vi "VI Anlagenuebersicht.vi"() -> (3 "XML-String":string)   [LabVIEW 2020, in "Anlagenuebersicht.lvlib"]
uses:
  VisBx Anzeige/Anlagenuebersicht.lvlib
  VisBx Anzeige/Messwerte.ctl
  PNS/Aktionen FGV Grenzwerte.ctl
  cRIO/PC/Kommunikation mit cRIO.lvlib
  Funktionstasten/Funktionstasten.lvlib
  Funktionstasten/Funktionstasten-Aktion.ctl
  Funktionstasten/Zustaende.ctl
  CalGas Aufschaltung/Auswahl Aufschaltpunkt.ctl
  CalGas Aufschaltung/CalGas Aufschaltung.lvlib
  CalGas Aufschaltung/FGV CalGas Aktionen.ctl
  PNS/PNS.lvlib
  PNS/Aktionen FGV Istwerte.ctl
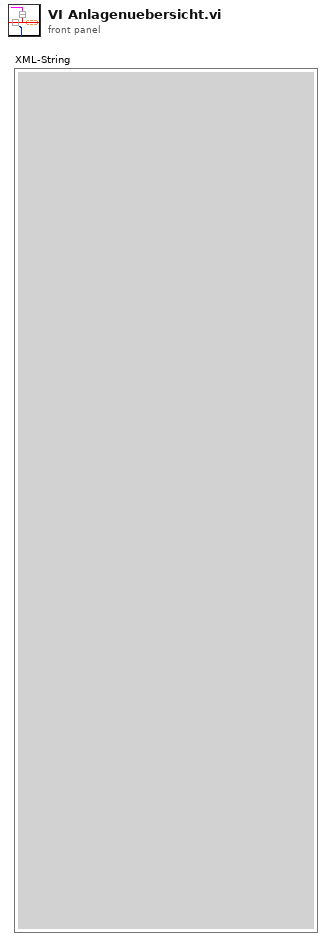
[diagram p1: front panel]
types:
  T1 = enum16{"Stby/Pause/Eco", "Messen", "Spülen Filter", "Spülen Leitung", "Umgebungsluft", "0-Gas / Hintergrund", "Cal-Gas"}
  T2 = typedef "Anlagenuebersicht.lvlib/Messwerte.ctl" = cluster{"-17S1":bool, "-17S2":bool, "-17S5":bool, "-17S6":bool, "-18B6":bool, "-16B1":bool, "-16B2":bool, "DI Reserve 1":bool, "DI Reserve 2":bool, "DI Reserve 3":bool, "DI Reserve 4":bool, "DI Reserve 5":bool, "-20Y1":bool, "-20Y2":bool, "-20Y3":bool, "-20Y4":bool, "-20Y5":bool, "-20Y6":bool, "-20Y7":bool, "-20Y8":bool, "-21Y1":bool, "-21Y2":bool, "-21Y3":bool, "-21Y4":bool, "-21Y5":bool, "-21Y6":bool, "-21Y7":bool, "-21Y8":bool, "-22Y1":bool, "-22Y2":bool, "-22Y3":bool, "-22Y4":bool, "-22Y5":bool, "-22Y6":bool, "-22Y7":bool, "-23Y1":bool, "-23Y2":bool, "-23Y3":bool, "-23Y4":bool, "-23Y5":bool, "-23Y6":bool, "-23Y7":bool, "Messgaspumpe EIN":bool, "Absaugung EIN":bool, "Kompressor":bool, "-23Y8":bool, "-11Y2":bool, "-11Y3":bool, "-11Y5":bool, "-11Y6":bool, "-11Y7":bool, "-11Y8":bool, "-12Y1":bool, "Zustand":enum16{"Stby/Pause/Eco", "Messen", "Spülen Filter", "Spülen Leitung", "Umgebungsluft", "0-Gas / Hintergrund", "Cal-Gas"}, "Reserve 1":bool, "Reserve 2":bool, "Reserve 3":bool, "Reserve 4":bool, "Reserve 5":bool, "Reserve 6":bool, "Reserve 7":bool, "Reserve 8":bool, "Reserve 9":bool, "Reserve 10":bool, "Reserve 11":bool, "Reserve 12":bool, "Reserve 13":bool, "Reserve 14":bool, "Reserve 15":bool, "Reserve 16":bool}
  T3 = typedef "CalGas Aufschaltung.lvlib/FGV CalGas Aktionen.ctl" = enum16{"lesen", "Analysator Auswahl", "Def.CalGas", "Aufschaltung CalGas", "laden", "speichern", "KAL extrahieren"}
  T4 = typedef "Funktionstasten.lvlib/Zustaende.ctl" = enum16{"Standby", "Pause", "Eco", "Messen", "Kalibrieren", "Spülen Filter", "Spülen Leitung", "Umgebungsluft", "0-Gas", "Cal-Gas", "CG zu PNS", "-------------", "Init 1", "Init 2", "Init 3", "Init 4", "Messen vorbereiten", "Messen durchführen", "Exit"}
  T5 = typedef "CalGas Aufschaltung.lvlib/Auswahl Aufschaltpunkt.ctl" = enum16{"über Filterblock", "Analysator direkt", "über PNS", "Entnahme", "Gasdivider"}
  T6 = typedef "Funktionstasten.lvlib/Funktionstasten-Aktion.ctl" = enum16{"Initialisieren", "Zustand setzen", "Taste gedrückt", "Fehler speichern", "Lesen", "Manuell", "Remote", "Bitparallel", "Samplepoint", "Zeit Prüfen", "reset Umschalten"}
  T7 = typedef "CalGas Aufschaltung.lvlib/Aufschaltung CalGas.ctl" = cluster{"Kalibriergas":T8, "Aufschaltpunkt":T5, "Analysator":T9}
  T8 = typedef "Auswahlfeld.ctl" = u16
  T9 = typedef "CalGas Aufschaltung.lvlib/Auswahl Analysator.ctl" = enum16{"FT-IR", "FID", "PMA", "PMA/FID/FT-IR"}
  T10 = typedef "PNS.lvlib/Aktionen FGV Istwerte.ctl" = enum16{"lesen", "initialisieren", "schreiben", "Störungen"}
  T11 = typedef "PNS.lvlib/Aktionen FGV Grenzwerte.ctl" = enum16{"lesen", "Grenzw. schreiben", "Anweisungscode", "IP-Adresse", "laden", "speichern", "Anweisungscode vorgeben"}
  T12 = typedef "Verwaltung - cRIO.lvlib/Digital Eingaenge 0-15.ctl" = cluster{"I0: N2 Nachf. FT-IR voll":bool, "I1: N2 Nachf. Vorrat leer":bool, "I2: (Klimaanlage eingeschaltet)":bool, "I3: (Klimaanlage Störung)":bool, "I4: Trigger Eingang (Messdaten sp.)":bool, "I5: Reserve":bool, "I6: Reserve":bool, "I7: Reserve":bool, "I8: Druckschalter Versorgung ok":bool, "I9: Reserve":bool, "I10: Reserve":bool, "I11: Reserve":bool, "I12: Drucksch. N2 Versorgung":bool, "I13: Reserve":bool, "I14: Drucksch. N2 Optikbox":bool, "I15: (Füllstand Kondensatbehälter)":bool}
  T13 = typedef "Verwaltung - cRIO.lvlib/Digital Ausgaenge 0-31.ctl" = cluster{"O0: Druckluft Versorgung":bool, "O1: CG 1 (FB Eingang 1)":bool, "O2: CG 2 (Kühlung FT-IR EIN)":bool, "O3: CG 3 (FB Bypass)":bool, "O4: CG 4 (FB CalGas)":bool, "O5: CG 5 (FB spülen/UL)":bool, "O6: CG 6 (FB zum FT-IR)":bool, "O7: CG 7 (FB zum FID)":bool, "O8: CG 8 (FB Reserve)":bool, "O9: (FB Reserve)":bool, "O10: (FB Umgebungsluft FID)":bool, "O11: (FB zum Gaskühler)":bool, "O12: FB Stickstoff zu FT-IR":bool, "O13: Optikbox FT-IR spülen":bool, "O14: (Purifier deaktivieren)":bool, "O15: (Umschaltung Purifier/Stickstoff)":bool, "O16: N2 Einblasung":bool, "O17: LSP LN2 Nachfüllung":bool, "O18: (Reserve)":bool, "O19: (Pumpe Eingang1)":bool, "O20: (Pumpe Eingang2)":bool, "O21: (Pumpe Spülen1)":bool, "O22: (Pumpe Spülen2)":bool, "O23: (Reserve)":bool, "O24: CalGas 1":bool, "O25: CalGas 2":bool, "O26: CG 3-8 (CalGas 3)":bool, "O27: Stickstoff aufschalten":bool, "O28: CG zu PNS":bool, "O29: FTIR Standby Spülung":bool, "O30: CG zu Entnahme(T90)":bool, "O31: (Purifier regenerieren)":bool}
  T14 = typedef "Verwaltung - cRIO.lvlib/Digital Ausgaenge 32-63.ctl" = cluster{"O32: Messgaspumpe EIN":bool, "O33: (Umgebungsluftpumpe)":bool, "O34: (Kondensatpumpe GK)":bool, "O35: Klima/Lüfter EIN":bool, "O36: Versorgung Heizungen":bool, "O37: Versorgung Heizungen":bool, "O38: (Gaskühler EIN (Freigabe))":bool, "O39: Störung FAS LP":bool, "O40: (Heizung Filterblock)":bool, "O41: Heizung HL zu FT-IR":bool, "O42: Heizung HL Extern SP1":bool, "O43: Heizung HL Extern SP2":bool, "O44: Heizung Reserve":bool, "O45: Heizung Reserve":bool, "O46: Statusbeleuchtung grün":bool, "O47: Statusbeleuchtung rot":bool}
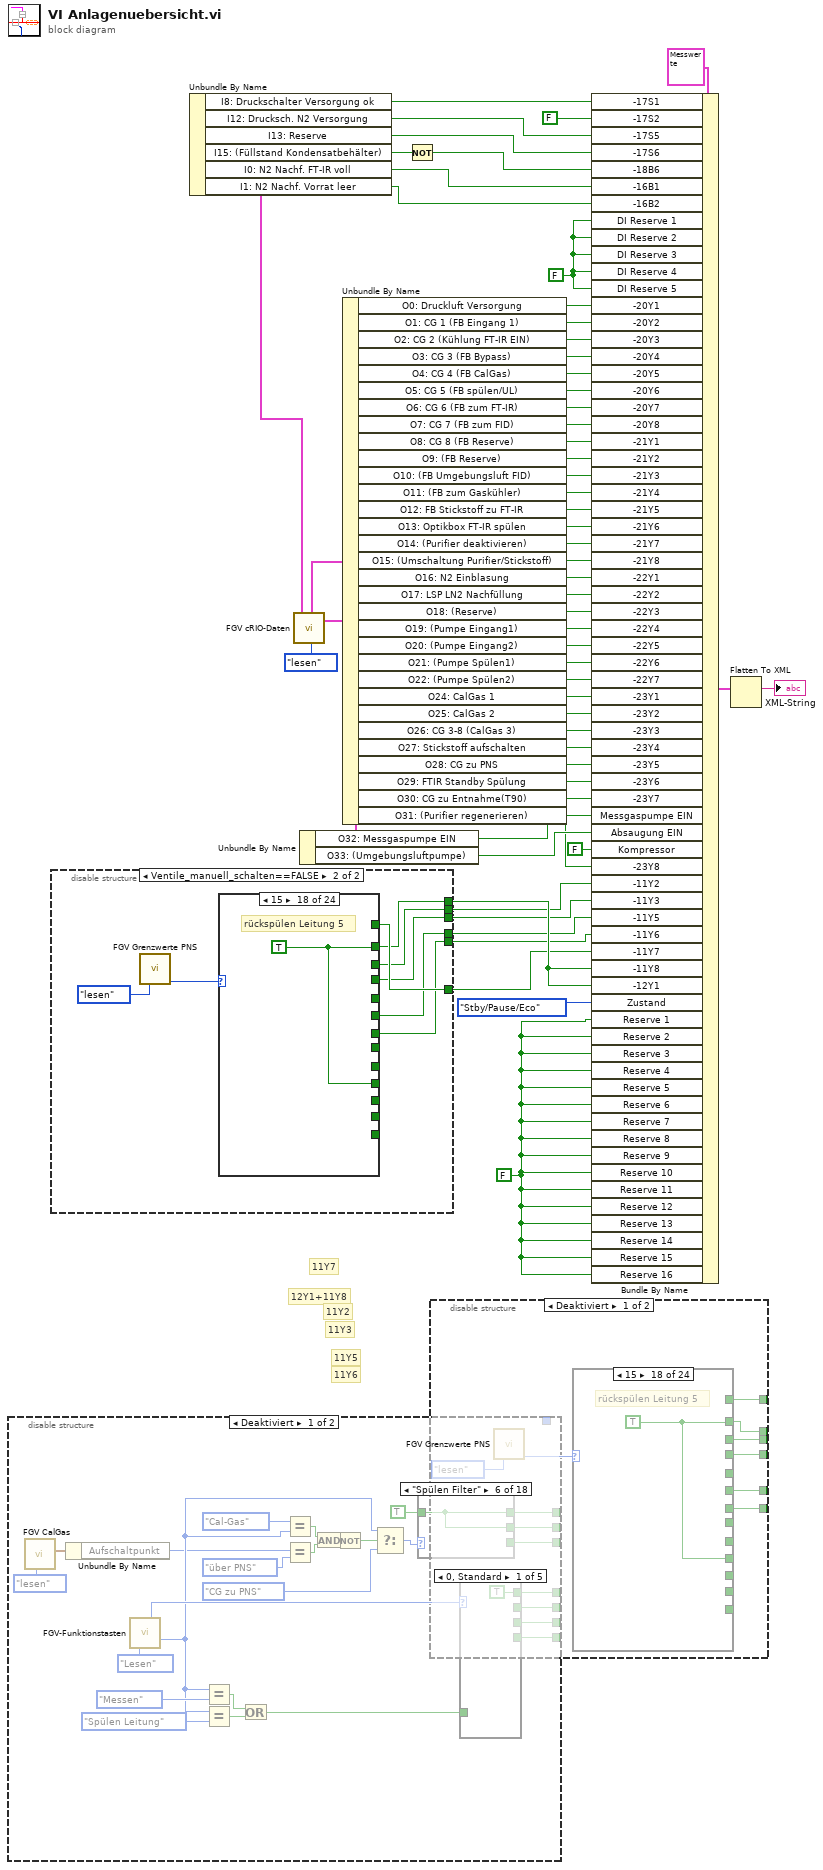
[diagram p0: block diagram]
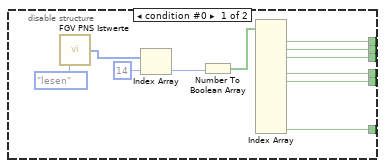
[diagram p2: hidden frame]
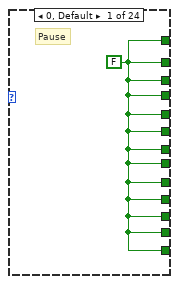
[diagram p3: hidden frame]
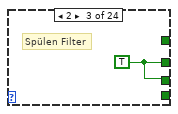
[diagram p5: hidden frame]
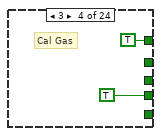
[diagram p6: hidden frame]
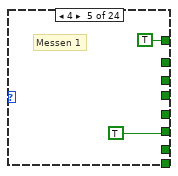
[diagram p7: hidden frame]
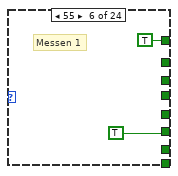
[diagram p8: hidden frame]
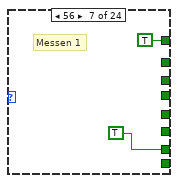
[diagram p9: hidden frame]
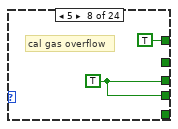
[diagram p10: hidden frame]
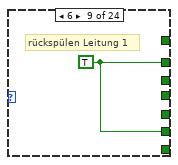
[diagram p11: hidden frame]
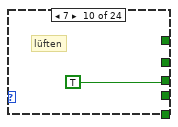
[diagram p12: hidden frame]
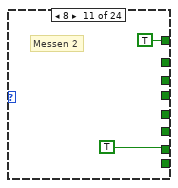
[diagram p13: hidden frame]
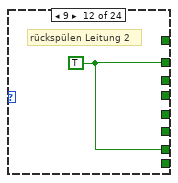
[diagram p14: hidden frame]
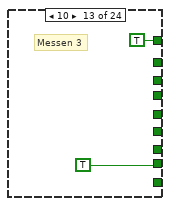
[diagram p15: hidden frame]
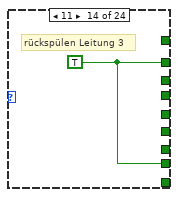
[diagram p16: hidden frame]
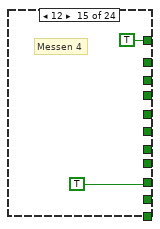
[diagram p17: hidden frame]
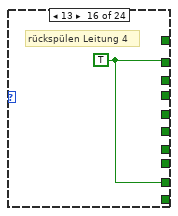
[diagram p18: hidden frame]
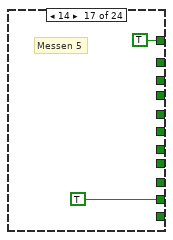
[diagram p19: hidden frame]
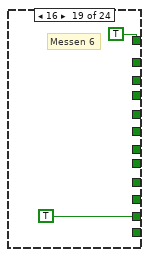
[diagram p20: hidden frame]
diagram:
  w7 = FALSE ("Reserve 11")
  w46 = FALSE ("DI Reserve 1")
  # "11Y6"
  # "11Y5"
  # "11Y3"
  # "11Y2"
  # "12Y1+11Y8"
  # "11Y7"
  n1 = disable-structure shown="Deaktiviert" {
    disable-tunnel: _ -> [w86 _]
    disable-tunnel: [w78 _] -> _
    disable-tunnel: [w77 _] -> _
    disable-tunnel: [w76 _] -> _
    disable-tunnel: [w75 _] -> _
    disable-tunnel: [w73 _] -> _
    disable-tunnel: [w72 _] -> _
    disable-tunnel: [w71 _] -> _
    frame Disabled {
      n2 = call "FGV CalGas.vi"("Aktionen"=FGV_CalGas_Aktionen."lesen") -> ("Aufschaltung CalGas"=w62:T7)  [unwired: 6 in, 4 out]
      n3 = Unbundle By Name(w62) -> ("Aufschaltpunkt"=w61:T5)
      n4 = call "FGV-Funktionstasten.vi"("Aktion"=Funktionstasten-Aktion."Lesen") -> ("Samplepoint"=w84:u16, "ausgewählte Funktion"=w63:T4)  [unwired: 7 in, 6 out]
      n5 = Equal?(x=w63, y=Zustaende."Messen" ("x")) -> (x = y?=w83:bool)
      n6 = Equal?(x=w63, y=Zustaende."Spülen Leitung" ("x")) -> (x = y?=w82:bool)
      n7 = Or(x=w83, y=w82) -> (x .or. y?=w81:bool)
      n8 = Equal?(x=Zustaende."Cal-Gas" ("y"), y=w63) -> (x = y?=w69:bool)
      n9 = Equal?(x=w61, y=Auswahl_Aufschaltpunkt."über PNS") -> (x = y?=w70:bool)
      n10 = And(x=w69, y=w70) -> (x .and. y?=w66:bool)
      n11 = Not(x=w66) -> (.not. x?=w60:bool)
      n12 = Select(t=w63, s=w60, f=Zustaende."CG zu PNS") -> (s? t:f=w64:T4)
      n13 = case shown="\"Spülen Filter\"" w64 {
        tunnel: TRUE -> [_ _ _ _ _ w87 w88 _ _ w89 _ _ _ _ _ _ _ _]
        tunnel: [_ _ _ _ _ w87 w88 _ _ _ _ _ _ _ _ _ _ _] -> w73
        tunnel: [_ _ _ _ _ w87 _ _ _ _ _ _ _ _ _ _ _ _] -> w72
        tunnel: [_ _ _ _ _ _ _ _ _ w89 _ _ _ _ _ _ _ _] -> w71
        frame "Standby", Default {
        }
        frame "Pause" {
        }
        frame "Eco" {
        }
        frame "Messen" {
        }
        frame "Kalibrieren" {
        }
        frame "Spülen Filter" {
        }
        frame "Spülen Leitung" {
        }
        frame "0-Gas" {
        }
        frame "Cal-Gas" {
        }
        frame "CG zu PNS" {
        }
        frame "-------------" {
        }
        frame "Init 1" {
        }
        frame "Init 2" {
        }
        frame "Init 3" {
        }
        frame "Init 4" {
        }
        frame "Messen vorbereiten" {
        }
        frame "Messen durchführen" {
        }
        frame "Exit" {
        }
      }
      n14 = case shown="0, Standard" w84 {
        tunnel: w81 -> [_ w91 w92 w93 w94]
        tunnel: [TRUE w91 _ _ _] -> w75
        tunnel: [_ _ w92 _ _] -> w76
        tunnel: [_ _ _ w93 _] -> w77
        tunnel: [_ _ _ _ w94] -> w78
        frame 0, Default {
        }
        frame 1 {
        }
        frame 2 {
        }
        frame 3 {
        }
        frame 4 {
        }
      }
    }
    frame Enabled {
    }
  }
  n15 = disable-structure shown="Ventile_manuell_schalten==FALSE" {
    disable-tunnel: [w100 w110] -> w6
    disable-tunnel: [w99 w109] -> w5
    disable-tunnel: [w98 w108] -> w4
    disable-tunnel: [w97 w107] -> w3
    disable-tunnel: [w96 w106] -> w2
    disable-tunnel: [w95 w111] -> w1
    frame condition #0 {
      n16 = call "FGV PNS Istwerte.vi"("Aktionen"=Aktionen_FGV_Istwerte."lesen") -> ("UsrVal"=w104:u16[])  [unwired: 11 in, 3 out]
      n17 = Index Array(array=w104, index=14 ("Index")) -> (element=w102:u16)
      n18 = Number To Boolean Array(number=w102) -> (Boolean array=w101:bool[])
      n19 = Index Array(array=w101) -> (element #1=w100:bool, element #2=w99:bool, element #3=w98:bool, element #5=w97:bool, element #6=w96:bool, element #12=w95:bool)  [unwired: 12 in, 6 out]
    }
    frame condition #1 (active) {
      n20 = call "FGV Grenzwerte PNS.vi"("Aktionen FGV Grenzwerte"=Aktionen_FGV_Grenzwerte."lesen") -> ("Anweisungscode"=w113:u16)  [unwired: 12 in, 2 out]
      n21 = case shown="15" w113 {
        tunnel: [w114 _ w115 _ _ _ _ _ w126 _ _ w130 _ w133 _ w136 _ w139 _ w142 _ w145 _ w148] -> w110
        tunnel: [w114 _ w115 _ _ _ _ w125 _ TRUE _ _ _ _ _ _ _ _ _ _ _ _ _ _] -> w109
        tunnel: [w114 _ _ TRUE _ _ _ w125 _ _ _ _ _ _ _ _ _ _ _ _ _ _ _ _] -> w108
        tunnel: [w114 _ _ _ _ _ _ _ _ _ _ _ _ _ _ _ _ _ _ _ _ _ _ _] -> _
        tunnel: [w114 _ _ _ TRUE TRUE _ _ w126 _ _ _ _ _ _ _ _ _ _ _ _ _ _ _] -> w107
        tunnel: [w114 _ _ _ _ _ TRUE _ _ _ TRUE w130 _ _ _ _ _ _ _ _ _ _ _ _] -> w106
        tunnel: [w114 _ _ _ _ _ _ _ _ _ _ _ TRUE w133 _ _ _ _ _ _ _ _ _ _] -> _
        tunnel: [w114 _ _ _ _ _ _ _ _ _ _ _ _ _ TRUE w136 _ _ _ _ _ _ _ _] -> _
        tunnel: [w114 _ _ _ _ _ _ _ _ _ _ _ _ _ _ _ TRUE w139 _ _ _ _ _ _] -> _
        tunnel: [w114 _ _ _ _ _ _ _ _ _ _ _ _ _ _ _ _ _ TRUE w142 _ _ _ _] -> _
        tunnel: [w114 _ _ _ _ _ _ _ _ _ _ _ _ _ _ _ _ _ _ _ TRUE w145 _ _] -> _
        tunnel: [w114 _ _ _ _ _ _ _ _ _ _ _ _ _ _ _ _ _ _ _ _ _ TRUE w148] -> _
        tunnel: [w114 _ _ TRUE TRUE TRUE TRUE TRUE _ _ TRUE _ TRUE _ TRUE _ TRUE _ TRUE _ TRUE _ TRUE _] -> w111
        frame 0, Default {
          w114 = FALSE
          # "Pause"
        }
        frame 1 {
          # "Standby"
        }
        frame 2 {
          w115 = TRUE
          # "Spülen Filter"
        }
        frame 3 {
          # "Cal Gas"
        }
        frame 4 {
          # "Messen 1"
        }
        frame 55 {
          # "Messen 1"
        }
        frame 56 {
          # "Messen 1"
        }
        frame 5 {
          w125 = TRUE
          # "cal gas overflow"
        }
        frame 6 {
          w126 = TRUE
          # "rückspülen Leitung 1"
        }
        frame 7 {
          # "lüften"
        }
        frame 8 {
          # "Messen 2"
        }
        frame 9 {
          w130 = TRUE
          # "rückspülen Leitung 2"
        }
        frame 10 {
          # "Messen 3"
        }
        frame 11 {
          w133 = TRUE
          # "rückspülen Leitung 3"
        }
        frame 12 {
          # "Messen 4"
        }
        frame 13 {
          w136 = TRUE
          # "rückspülen Leitung 4"
        }
        frame 14 {
          # "Messen 5"
        }
        frame 15 {
          w139 = TRUE
          # "rückspülen Leitung 5"
        }
        frame 16 {
          # "Messen 6"
        }
        frame 17 {
          w142 = TRUE
          # "rückspülen Leitung 6"
        }
        frame 18 {
          # "Messen 7"
        }
        frame 19 {
          w145 = TRUE
          # "rückspülen Leitung 7"
        }
        frame 20 {
          # "Messen 8"
        }
        frame 21 {
          w148 = TRUE
          # "rückspülen Leitung 8"
        }
      }
    }
  }
  n22 = call "FGV cRIO-Daten.vi"("Aktion"=enum16{"lesen", "schreiben"}."lesen") -> ("DI"=w54:T12, "DO 0-31"=w53:T13, "DO 32-63"=w52:T14)  [unwired: 9 in, 7 out]
  n23 = Unbundle By Name(w54) -> ("I8: Druckschalter Versorgung ok"=w51:bool, "I12: Drucksch. N2 Versorgung"=w50:bool, "I13: Reserve"=w49:bool, "I15: (Füllstand Kondensatbehälter)"=w48:bool, "I0: N2 Nachf. FT-IR voll"=w13:bool, "I1: N2 Nachf. Vorrat leer"=w12:bool)
  n24 = Unbundle By Name(w52) -> ("O32: Messgaspumpe EIN"=w16:bool, "O33: (Umgebungsluftpumpe)"=w15:bool)
  n25 = Unbundle By Name(w53) -> ("O0: Druckluft Versorgung"=w45:bool, "O1: CG 1 (FB Eingang 1)"=w44:bool, "O2: CG 2 (Kühlung FT-IR EIN)"=w43:bool, "O3: CG 3 (FB Bypass)"=w42:bool, "O4: CG 4 (FB CalGas)"=w41:bool, "O5: CG 5 (FB spülen/UL)"=w40:bool, "O6: CG 6 (FB zum FT-IR)"=w11:bool, "O7: CG 7 (FB zum FID)"=w39:bool, "O8: CG 8 (FB Reserve)"=w38:bool, "O9: (FB Reserve)"=w37:bool, "O10: (FB Umgebungsluft FID)"=w36:bool, "O11: (FB zum Gaskühler)"=w35:bool, "O12: FB Stickstoff zu FT-IR"=w34:bool, "O13: Optikbox FT-IR spülen"=w33:bool, "O14: (Purifier deaktivieren)"=w32:bool, "O15: (Umschaltung Purifier/Stickstoff)"=w31:bool, "O16: N2 Einblasung"=w30:bool, "O17: LSP LN2 Nachfüllung"=w29:bool, "O18: (Reserve)"=w28:bool, "O19: (Pumpe Eingang1)"=w27:bool, "O20: (Pumpe Eingang2)"=w26:bool, "O21: (Pumpe Spülen1)"=w25:bool, "O22: (Pumpe Spülen2)"=w24:bool, "O24: CalGas 1"=w17:bool, "O25: CalGas 2"=w18:bool, "O26: CG 3-8 (CalGas 3)"=w19:bool, "O27: Stickstoff aufschalten"=w20:bool, "O28: CG zu PNS"=w21:bool, "O29: FTIR Standby Spülung"=w22:bool, "O30: CG zu Entnahme(T90)"=w23:bool, "O31: (Purifier regenerieren)"=w10:bool)
  n26 = Not(x=w48) -> (.not. x?=w47:bool)
  n27 = disable-structure shown="Deaktiviert" {
    disable-tunnel: [w154 _] -> _
    disable-tunnel: [w153 _] -> _
    disable-tunnel: [w152 _] -> _
    disable-tunnel: [w151 _] -> _
    disable-tunnel: [w150 _] -> _
    disable-tunnel: [w149 _] -> _
    frame Disabled {
      n28 = call "FGV Grenzwerte PNS.vi"("Aktionen FGV Grenzwerte"=Aktionen_FGV_Grenzwerte."lesen") -> ("Anweisungscode"=w155:u16)  [unwired: 12 in, 2 out]
      n29 = case shown="15" w155 {
        tunnel: [w157 _ w158 _ _ _ _ _ w169 _ _ w173 _ w176 _ w179 _ w182 _ w185 _ w188 _ w191] -> w152
        tunnel: [w157 _ w158 _ _ _ _ w168 _ TRUE _ _ _ _ _ _ _ _ _ _ _ _ _ _] -> w151
        tunnel: [w157 _ _ TRUE _ _ _ w168 _ _ _ _ _ _ _ _ _ _ _ _ _ _ _ _] -> w149
        tunnel: [w157 _ _ _ _ _ _ _ _ _ _ _ _ _ _ _ _ _ _ _ _ _ _ _] -> _
        tunnel: [w157 _ _ _ TRUE TRUE _ _ w169 _ _ _ _ _ _ _ _ _ _ _ _ _ _ _] -> w154
        tunnel: [w157 _ _ _ _ _ TRUE _ _ _ TRUE w173 _ _ _ _ _ _ _ _ _ _ _ _] -> w153
        tunnel: [w157 _ _ _ _ _ _ _ _ _ _ _ TRUE w176 _ _ _ _ _ _ _ _ _ _] -> _
        tunnel: [w157 _ _ _ _ _ _ _ _ _ _ _ _ _ TRUE w179 _ _ _ _ _ _ _ _] -> _
        tunnel: [w157 _ _ _ _ _ _ _ _ _ _ _ _ _ _ _ TRUE w182 _ _ _ _ _ _] -> _
        tunnel: [w157 _ _ _ _ _ _ _ _ _ _ _ _ _ _ _ _ _ TRUE w185 _ _ _ _] -> _
        tunnel: [w157 _ _ _ _ _ _ _ _ _ _ _ _ _ _ _ _ _ _ _ TRUE w188 _ _] -> _
        tunnel: [w157 _ _ _ _ _ _ _ _ _ _ _ _ _ _ _ _ _ _ _ _ _ TRUE w191] -> _
        tunnel: [w157 _ _ TRUE TRUE TRUE TRUE TRUE _ _ TRUE _ TRUE _ TRUE _ TRUE _ TRUE _ TRUE _ TRUE _] -> w150
        frame 0, Default {
          w157 = FALSE
          # "Pause"
        }
        frame 1 {
          # "Standby"
        }
        frame 2 {
          w158 = TRUE
          # "Spülen Filter"
        }
        frame 3 {
          # "Cal Gas"
        }
        frame 4 {
          # "Messen 1"
        }
        frame 55 {
          # "Messen 1"
        }
        frame 56 {
          # "Messen 1"
        }
        frame 5 {
          w168 = TRUE
          # "cal gas overflow"
        }
        frame 6 {
          w169 = TRUE
          # "rückspülen Leitung 1"
        }
        frame 7 {
          # "lüften"
        }
        frame 8 {
          # "Messen 2"
        }
        frame 9 {
          w173 = TRUE
          # "rückspülen Leitung 2"
        }
        frame 10 {
          # "Messen 3"
        }
        frame 11 {
          w176 = TRUE
          # "rückspülen Leitung 3"
        }
        frame 12 {
          # "Messen 4"
        }
        frame 13 {
          w179 = TRUE
          # "rückspülen Leitung 4"
        }
        frame 14 {
          # "Messen 5"
        }
        frame 15 {
          w182 = TRUE
          # "rückspülen Leitung 5"
        }
        frame 16 {
          # "Messen 6"
        }
        frame 17 {
          w185 = TRUE
          # "rückspülen Leitung 6"
        }
        frame 18 {
          # "Messen 7"
        }
        frame 19 {
          w188 = TRUE
          # "rückspülen Leitung 7"
        }
        frame 20 {
          # "Messen 8"
        }
        frame 21 {
          w191 = TRUE
          # "rückspülen Leitung 8"
        }
      }
    }
    frame Enabled {
      # "11Y6"
      # "11Y5"
      # "11Y3"
      # "11Y2"
      # "12Y1+11Y8"
      # "11Y7"
    }
  }
  n30 = Bundle By Name(cluster=T2 {"-17S1"=FALSE, "-17S2"=FALSE, "-17S5"=FALSE, "-17S6"=FALSE, "-18B6"=FALSE, "-16B1"=FALSE, "-16B2"=FALSE, "DI Reserve 1"=FALSE, "DI Reserve 2"=FALSE, "DI Reserve 3"=FALSE, "DI Reserve 4"=FALSE, "DI Reserve 5"=FALSE, "-20Y1"=FALSE, "-20Y2"=FALSE, "-20Y3"=FALSE, "-20Y4"=FALSE, "-20Y5"=FALSE, "-20Y6"=FALSE, "-20Y7"=FALSE, "-20Y8"=FALSE, "-21Y1"=FALSE, "-21Y2"=FALSE, "-21Y3"=FALSE, "-21Y4"=FALSE, "-21Y5"=FALSE, "-21Y6"=FALSE, "-21Y7"=FALSE, "-21Y8"=FALSE, "-22Y1"=FALSE, "-22Y2"=FALSE, "-22Y3"=FALSE, "-22Y4"=FALSE, "-22Y5"=FALSE, "-22Y6"=FALSE, "-22Y7"=FALSE, "-23Y1"=FALSE, "-23Y2"=FALSE, "-23Y3"=FALSE, "-23Y4"=FALSE, "-23Y5"=FALSE, "-23Y6"=FALSE, "-23Y7"=FALSE, "Messgaspumpe EIN"=FALSE, "Absaugung EIN"=FALSE, "Kompressor"=FALSE, "-23Y8"=FALSE, "-11Y2"=FALSE, "-11Y3"=FALSE, "-11Y5"=FALSE, "-11Y6"=FALSE, "-11Y7"=FALSE, "-11Y8"=FALSE, "-12Y1"=FALSE, "Zustand"=enum."Stby/Pause/Eco", "Reserve 1"=FALSE, "Reserve 2"=FALSE, "Reserve 3"=FALSE, "Reserve 4"=FALSE, "Reserve 5"=FALSE, "Reserve 6"=FALSE, "Reserve 7"=FALSE, "Reserve 8"=FALSE, "Reserve 9"=FALSE, "Reserve 10"=FALSE, "Reserve 11"=FALSE, "Reserve 12"=FALSE, "Reserve 13"=FALSE, "Reserve 14"=FALSE, "Reserve 15"=FALSE, "Reserve 16"=FALSE} ("Messwerte"), "-17S1"=w51, "-17S2"=FALSE, "-17S5"=w50, "-17S6"=w49, "-18B6"=w47, "-16B1"=w13, "-16B2"=w12, "DI Reserve 1"=w46, "DI Reserve 2"=w46, "DI Reserve 3"=w46, "DI Reserve 4"=w46, "DI Reserve 5"=w46, "-20Y1"=w45, "-20Y2"=w44, "-20Y3"=w43, "-20Y4"=w42, "-20Y5"=w41, "-20Y6"=w40, "-20Y7"=w11, "-20Y8"=w39, "-21Y1"=w38, "-21Y2"=w37, "-21Y3"=w36, "-21Y4"=w35, "-21Y5"=w34, "-21Y6"=w33, "-21Y7"=w32, "-21Y8"=w31, "-22Y1"=w30, "-22Y2"=w29, "-22Y3"=w28, "-22Y4"=w27, "-22Y5"=w26, "-22Y6"=w25, "-22Y7"=w24, "-23Y1"=w17, "-23Y2"=w18, "-23Y3"=w19, "-23Y4"=w20, "-23Y5"=w21, "-23Y6"=w22, "-23Y7"=w23, "Messgaspumpe EIN"=w16, "Absaugung EIN"=w15, "Kompressor"=FALSE, "-23Y8"=w10, "-11Y2"=w5, "-11Y3"=w4, "-11Y5"=w3, "-11Y6"=w2, "-11Y7"=w1, "-11Y8"=w6, "-12Y1"=w6, "Zustand"=T1."Stby/Pause/Eco", "Reserve 1"=w7, "Reserve 2"=w7, "Reserve 3"=w7, "Reserve 4"=w7, "Reserve 5"=w7, "Reserve 6"=w7, "Reserve 7"=w7, "Reserve 8"=w7, "Reserve 9"=w7, "Reserve 10"=w7, "Reserve 11"=w7, "Reserve 12"=w7, "Reserve 13"=w7, "Reserve 14"=w7, "Reserve 15"=w7, "Reserve 16"=w7) -> (w58:T2)
  n31 = Flatten To XML(6:w58) -> (2:→"XML-String":string)
